vi "Lab.04_DAQ.vi"() -> ()   [LabVIEW 2016]
uses:
  <vilib>/Analysis/2dsp.llb/Real FFT.vi
  <vilib>/Analysis/2dsp.llb/Power Spectrum (DBL).vi
  <vilib>/Analysis/NI_AALPro.lvlib
panel:
  out "Boolean":bool
  out "Numeric":dbl
  out "Min":dbl
  out "Max":dbl
  out "channel B":dynamicdata(graph)
  out "channel A":dynamicdata(graph)
  out "Fourier Transformation":dbl[](graph)
  out "FFT(X)":cdb[](array[numeric])
  out "Added signals":dynamicdata(graph)
  out "Filtered signals":dynamicdata(graph)
  in  "stop":bool
  out "Input signals":dynamicdata(graph)
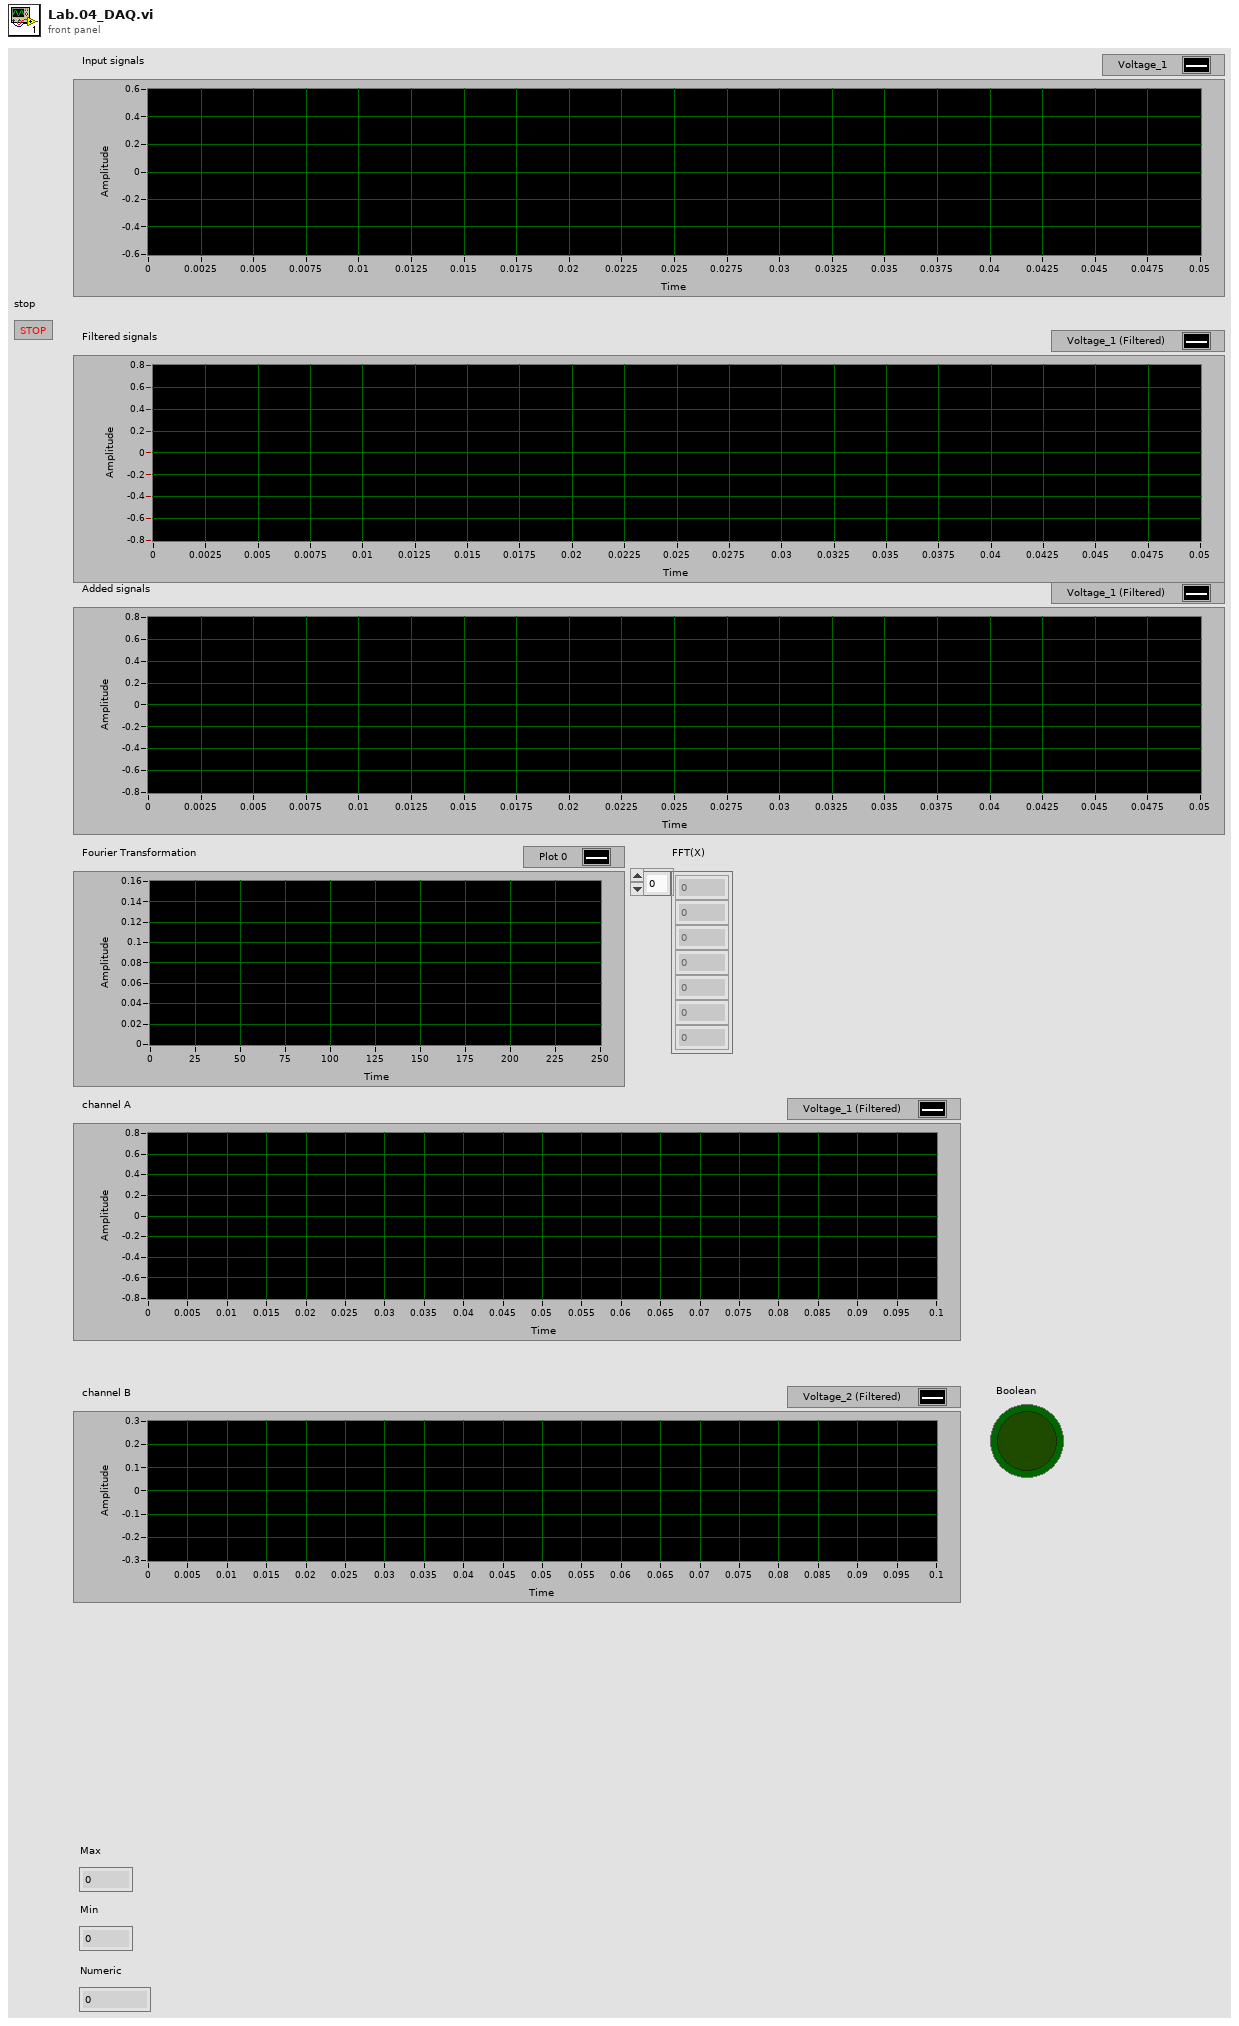
[diagram p1: front panel]
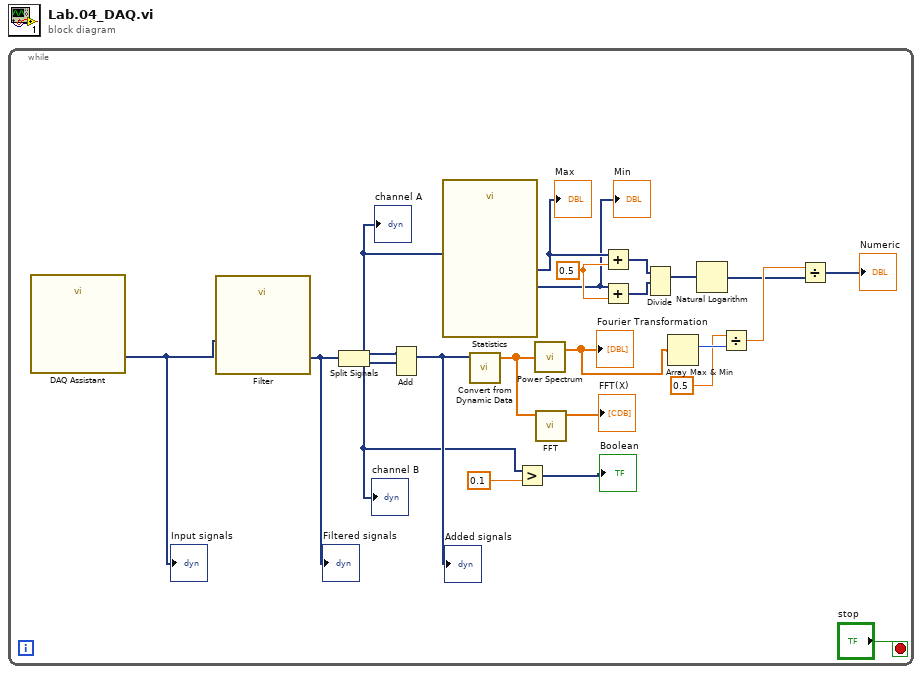
[diagram p0: block diagram]
diagram:
  n1 = while {
    stop <- "stop" stop-if-true
    w6 = 0.5
    n2 = call "DAQ Assistant"() -> ("data"=w17:dynamicdata)  [unwired: 16 in, 3 out]
    "Input signals" <- w17
    n3 = call "Filter"("Signal"=w17) -> ("Filtered Signal"=w21:dynamicdata)  [unwired: 9 in, 1 out]
    "Filtered signals" <- w21
    n4 = Split Signals(w21) -> (w3:dynamicdata, w2:dynamicdata)  [unwired: 2 in]
    "channel A" <- w3
    "channel B" <- w2
    n5 = Add(1:w2, 2:w3) -> (0:w20:dynamicdata)  [unwired: 1 in, 1 out]
    "Added signals" <- w20
    n6 = call "Statistics"("Signals"=w3) -> ("Minimum"=w5:dynamicdata, "Maximum"=w7:dynamicdata)  [unwired: 22 in, 3 out]
    "Max" <- w7
    "Min" <- w5
    n7 = call "Convert from Dynamic Data"("Dynamic Data Type"=w20) -> ("Array"=w19:dbl[])  [unwired: 3 in]
    n8 = Greater?(x=w2, y=0.1) -> (0:→"Boolean":dynamicdata)
    n9 = call-poly <vilib>:"Power Spectrum.vi"("X"=w19) -> ("Power Spectrum"=w15:dbl[])  [unwired: 1 out]
    "Fourier Transformation" <- w15
    n10 = call-poly <vilib>:"FFT.vi"("X"=w19) -> ("FFT {X}"=→"FFT(X)":cdb[])  [unwired: 9 in, 1 out]
    n11 = Add(x=w7, y=w6) -> (x+y=w8:dynamicdata)
    n12 = Add(x=w5, y=w6) -> (x+y=w9:dynamicdata)
    n13 = Divide(1:w9, 2:w8) -> (0:w16:dynamicdata)  [unwired: 1 in, 1 out]
    n14 = Array Max & Min(array=w15) -> (max index (indices)=w14:i32)  [unwired: 3 out]
    n15 = Natural Logarithm(1:w16) -> (0:w11:dynamicdata)
    n16 = Divide(x=0.5, y=w14) -> (x/y=w12:dbl)
    n17 = Divide(x=w12, y=w11) -> (x/y=→"Numeric":dynamicdata)
  }
